vi "Homography UnitX.vi"() -> ()   [LabVIEW 2015]
uses:
  CalibrationCoordinates.vi
  <vilib>/Analysis/Matrix/NI_Matrix.lvlib
  <vilib>/Analysis/Matrix/Numeric/Conversions/Matrix To Array - RM.vi
panel:
  out "XY Graph":cluster{dbl, dbl}[](graph)
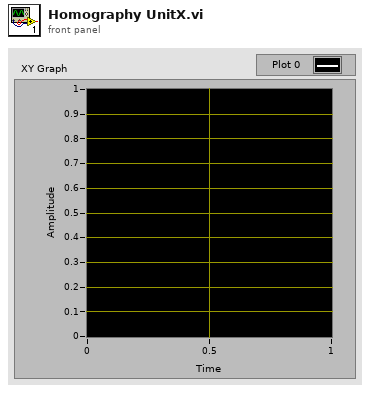
[diagram p1: front panel]
types:
  T1 = cluster{"Top Left":dbl[], "Top Right":dbl[], "Bottom Left":dbl[], "Bottom Right":dbl[]}
  T2 = typedef "NI_Matrix.lvlib/RealMatrix.ctl" = dbl[][]
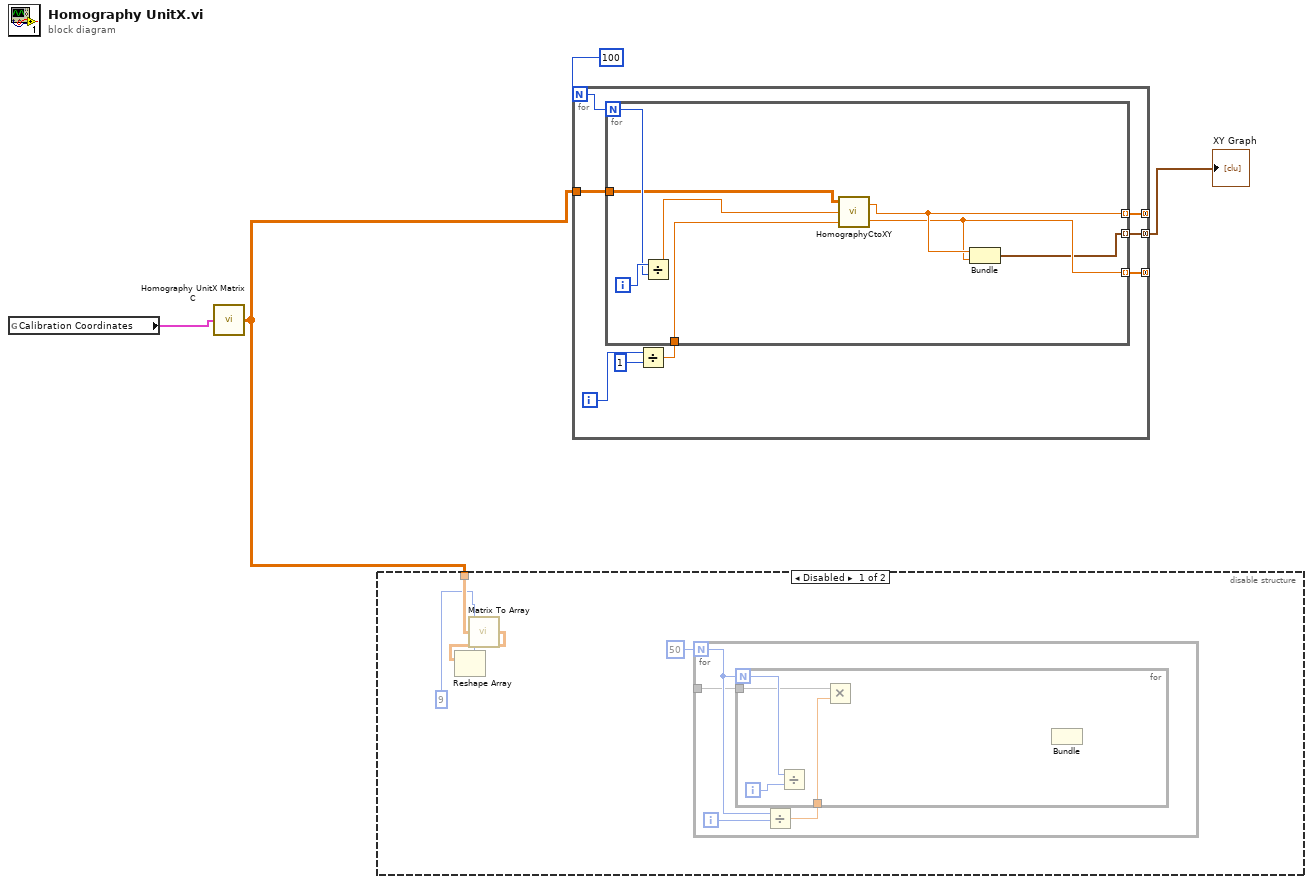
[diagram p0: block diagram]
diagram:
  n1 = global read "CalibrationCoordinates.vi" "Calibration Coordinates"() -> (w2:T1)
  n2 = call "Homography UnitX Matrix C.vi"("input cluster"=w2) -> ("C"=w1:T2)
  n3 = disable-structure shown="Disabled" {
    disable-tunnel: w1 -> [w10 _]
    frame Disabled {
      n4 = call-poly <vilib>:"Matrix To Array.vi"("Real Matrix"=w10) -> ("Real 2D Array"=w9:dbl[][])
      n5 = Reshape Array(w9, 9 ("dimension size")) -> (w8:dbl[])
      n6 = for {
        N: 50 -> [w13]
        tunnel: [w12] -> w6
        i -> [w14]
        n7 = Divide(x=w13, y=w14) -> (x/y=w11:dbl)
        n8 = for {
          N: w13 -> [w17]
          tunnel: w12 -> [w16]
          tunnel: w11 -> [w15]
          i -> [w18]
          n9 = Divide(x=w17, y=w18) -> ()  [unwired: 1 out]
          n10 = Multiply(x=w16, y=w15) -> ()  [unwired: 1 out]
          n11 = Bundle() -> ()  [unwired: 3 in, 1 out]
        }
      }
    }
    frame Enabled {
    }
  }
  n12 = for {
    N: 100 ("y") -> [w22]
    tunnel: w1 -> [w26]
    tunnel: [w23] -> w3 mode=concatenating
    tunnel: [w21] -> _ mode=concatenating
    tunnel: [w20] -> _ mode=concatenating
    i -> [w25]
    n13 = Divide(x=w25, y=1) -> (x/y=w24:dbl)
    n14 = for {
      N: w22 -> [w33]
      tunnel: w26 -> [w32]
      tunnel: w24 -> [w30]
      tunnel: [w27] -> w23 mode=indexing
      tunnel: [w28] -> w21 mode=indexing
      tunnel: [w29] -> w20 mode=indexing
      i -> [w34]
      n15 = Divide(x=w34, y=w33) -> (x/y=w31:dbl)
      n16 = call "HomographyCtoXY.vi"("Y"=w30, "X"=w31, "C"=w32) -> ("Y"=w28:dbl, "X"=w29:dbl)
      n17 = Bundle("X"=w29, "Y"=w28) -> (w27:cluster{"X":dbl, "Y":dbl})  [unwired: 1 in]
    }
  }
  "XY Graph" <- w3
